vi "ActionVIOnDelete.vi"(6 "All deleted Refs":T1[](array[typedef]) format="%.0x", 8 "error in (no error)":errorcluster, 11 "Item Ref in":T1 format="%.0x") -> (0 "error out":errorcluster, 3 "Item Ref out":T1 format="%.0x")   [LabVIEW 2016, in "PXImc Custom Device System Explorer.lvlib"]
uses:
  PXImc Custom Device System Explorer.lvlib
  <vilib>/NI Veristand/Custom Device API/Custom Device Item Ref.ctl
  Shared/Compiled.Settings.ctl
  PXImc Router/Controls/Target Type.ctl
  PXImc Router/Controls/Router - Configuration.ctl
  PXImc Router/Controls/Router/Node Block R-W Properties.ctl
  PXImc Router/Controls/Router/Block Properties.ctl
  PXImc Router/Controls/Router/Router - PXImc Properties.ctl
  PXImc Router/Controls/Router/Router - PXImc Card Properties.ctl
  PXImc Router/Controls/Node Data.ctl
  PXImc Router/Controls/Node/Node - PXImc Parameters.ctl
  PXImc Router/Controls/Node/Node - Writer Data.ctl
  <vilib>/NI Veristand/VeriStand Data/Byte Buffer/Byte Buffer.lvclass
  PXImc Router/Controls/Node/Node Ch Properties.ctl
  PXImc Router/Controls/Data Type.ctl
  PXImc Router/Controls/Node/Node - Readers Data.ctl
  PXImc Router/Controls/Node/Node - Reader Data.ctl
  Shared/Constants.vi
  <vilib>/NI Veristand/Custom Device Tools/Custom Device Utility Library/NI VeriStand - Search for Item by Name.vi
  <vilib>/NI Veristand/Custom Device API/Get Item Property (Variant).vi
  <vilib>/Utility/file.llb/Read Delimited Spreadsheet (string).vi
  <vilib>/Utility/file.llb/Write Delimited Spreadsheet (string).vi
  Shared/PXImc Custom Device Shared.lvlib
  <vilib>/NI VeriStand/Custom Device API/Custom Device API.lvlib
  PXImc Router/PXImc Router.lvlib
  <vilib>/NI VeriStand/Custom Device Tools/Custom Device Utility Library/Custom Device Utility Library.lvlib
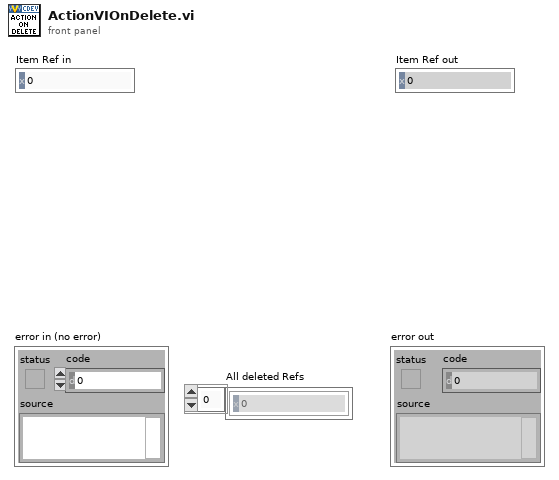
[diagram p1: front panel]
types:
  T1 = typedef "Custom Device API.lvlib/Custom Device Item Ref.ctl" = u64
  T2 = typedef "PXImc Custom Device Shared.lvlib/Compiled.Settings.ctl" = cluster{"Target Type":T3, "Router Properties":T4, "Node Data":T9, "Configuration Folder Path":path}
  T3 = typedef "PXImc Router.lvlib/Target Type.ctl" = enum16{"Router", "Node"}
  T4 = typedef "PXImc Router.lvlib/Router - Configuration.ctl" = cluster{"Target Type":T3, "Master Table Ref":refnum<data-value>, "Master Table Size (Bytes)":u32, "Node Properties":T5[], "Router - PXImc Properties":T7}
  T5 = typedef "PXImc Router.lvlib/Node Block R-W Properties.ctl" = cluster{"Node ID":u32, "# Reading Blocks":u32, "Node Writing Block":T6, "Node Reading Blocks":T6[]}
  T6 = typedef "PXImc Router.lvlib/Block Properties.ctl" = cluster{"Offset":u32, "Size (Bytes)":u32}
  T7 = typedef "PXImc Router.lvlib/Router - PXImc Properties.ctl" = cluster{"PXImc Cards Properties":T8[], "Connection Timeout (s)":dbl, "Readers Buffer Size":u64}
  T8 = typedef "PXImc Router.lvlib/Router - PXImc Card Properties.ctl" = cluster{"PXImc Resource Name":string, "Reader - PXImc Session Ref":refnum<k21>, "Writer - PXImc Session Ref":refnum<k21>, "Reader Conn ID":u16, "Writer Conn ID":u16}
  T9 = typedef "PXImc Router.lvlib/Node Data.ctl" = cluster{"Node Name":string, "PXImc Parameters":T10, "Local Data":T11, "Imported Data":T14}
  T10 = typedef "PXImc Router.lvlib/Node - PXImc Parameters.ctl" = cluster{"Resource Name":string, "Connection Timeout (s)":dbl, "Readers Buffer Size":u64, "Node PXImc Reader Conn Id":u16, "Node PXImc Writer Conn Id":u16, "Writer PXImc Session":refnum<k21>, "Reader PXImc Session":refnum<k21>}
  T11 = typedef "PXImc Router.lvlib/Node - Writer Data.ctl" = cluster{"Noder ID":u32, "Byte Buffer Ref":refnum<class "Byte Buffer.lvclass">, "Master Table Offest":u32, "Byte Buffer Size":u32, "Node Local Channels":T12[], "Node Local Channels Table":string[][]}
  T12 = typedef "PXImc Router.lvlib/Node Ch Properties.ctl" = cluster{"Name":string, "Value":dbl, "Data Type":T13}
  T13 = typedef "PXImc Router.lvlib/Data Type.ctl" = enum16{"Boolean", "SGL", "DBL", "I8", "I16", "I32", "I64", "U8", "U16", "U32", "U64"}
  T14 = typedef "PXImc Router.lvlib/Node - Readers Data.ctl" = cluster{"Byte Buffer Ref":refnum<class "Byte Buffer.lvclass">, "Byte Buffer Size":u64, "Readers Data Array":T15[], "Node Imported Channels Table":string[][]}
  T15 = typedef "PXImc Router.lvlib/Node - Reader Data.ctl" = cluster{"Noder ID":u32, "Master Table Offest":u32, "Byte Buffer Size":u64, "Node Imported Channels":T12[]}
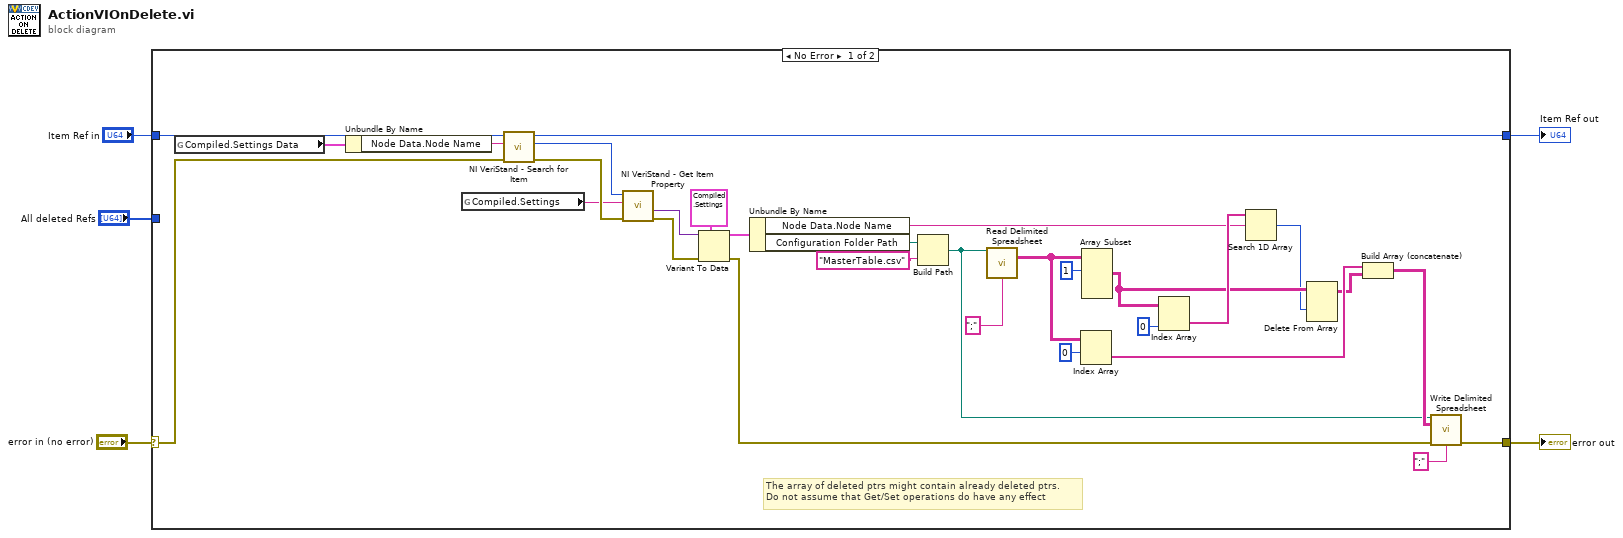
[diagram p0: block diagram]
diagram:
  n1 = case shown="No Error" "error in (no error)" {
    selector: "error in (no error)" -> [w7 w37]
    tunnel: [w14 w37] -> w4
    tunnel: "Item Ref in" -> [w11 w36]
    tunnel: [w6 w36] -> w2
    tunnel: "All deleted Refs" -> [_ _]
    frame No Error {
      # "The array of deleted ptrs might contain already deleted ptrs.\nDo not assume that Get/Set operations do have any effect"
      n2 = global read "Constants.vi" "Compiled.Settings Data"() -> (w13:T2)
      n3 = Unbundle By Name(w13) -> ("Node Data.Node Name"=w12:string)
      n4 = global read "Constants.vi" "Compiled.Settings"() -> (w8:string)
      n5 = call-poly <vilib>:"NI VeriStand - Search for Item.vi"("error in"=w7, "Item Name"=w12, "Section Ref in"=w11) -> ("error out"=w9:errorcluster, "Item Ref"=w10:T1, "Section Ref out"=w6:T1)  [unwired: 5 in, 1 out]
      n6 = call-poly <vilib>:"NI VeriStand - Get Item Property.vi"("error in (no error)"=w9, "Property Name"=w8, "Item Ref in"=w10) -> ("error out"=w28:errorcluster, "Value"=w30:variant)  [unwired: 5 in, 2 out]
      n7 = Variant To Data(error in=w28, type=T2 {"Target Type"=enum."Router", "Router Properties"={"Target Type"=enum."Router", "Master Table Ref"=refnum, "Master Table Size (Bytes)"=0, "Node Properties"=[], "Router - PXImc Properties"={"PXImc Cards Properties"=[], "Connection Timeout (s)"=0.0, "Readers Buffer Size"=0}}, "Node Data"={"Node Name"="", "PXImc Parameters"={"Resource Name"="", "Connection Timeout (s)"=0.0, "Readers Buffer Size"=0, "Node PXImc Reader Conn Id"=0, "Node PXImc Writer Conn Id"=0, "Writer PXImc Session"="", "Reader PXImc Session"=""}, "Local Data"={"Noder ID"=0, "Byte Buffer Ref"=refnum, "Master Table Offest"=0, "Byte Buffer Size"=0, "Node Local Channels"=[], "Node Local Channels Table"=[]}, "Imported Data"={"Byte Buffer Ref"=refnum, "Byte Buffer Size"=0, "Readers Data Array"=[], "Node Imported Channels Table"=[]}}, "Configuration Folder Path"=path ""} ("Compiled.Settings"), Variant=w30) -> (data=w29:T2, error out=w15:errorcluster)
      n8 = Unbundle By Name(w29) -> ("Node Data.Node Name"=w23:string, "Configuration Folder Path"=w34:path)
      n9 = Build Path(base path=w34, name or relative path="MasterTable.csv") -> (appended path=w16:path)
      n10 = call-poly <vilib>:"Read Delimited Spreadsheet.vi"("file path (dialog if empty)"=w16, "delimiter (\\t)"=";" ("delimiter (\\t)")) -> ("all rows"=w27:string[][])  [unwired: 8 in, 5 out]
      n11 = Index Array(array=w27, index (row)=0) -> (element=w20:string[])  [unwired: 1 in]
      n12 = Array Subset(array=w27, index (row)=1 ("index")) -> (w22:string[][])  [unwired: 3 in]
      n13 = Index Array(array=w22, index (col)=0 ("disabled index (col)")) -> (element=w24:string[])  [unwired: 1 in]
      n14 = Search 1D Array(1D array=w24, element=w23) -> (index of element=w21:i32)  [unwired: 1 in]
      n15 = Delete From Array(array=w22, index (row)=w21) -> (array with subset deleted=w19:string[][])  [unwired: 2 in, 1 out]
      n16 = Build Array (concatenate)(w20, w19) -> (w17:string[][])
      n17 = call-poly <vilib>:"Write Delimited Spreadsheet.vi"("file path (dialog if empty)"=w16, "2D data"=w17, "error in (no error)"=w15, "delimiter (\\t)"=";" ("delimiter (\\t)")) -> ("error out"=w14:errorcluster)  [unwired: 10 in, 1 out]
    }
    frame Error {
    }
  }
  "error out" <- w4
  "Item Ref out" <- w2
